vi "mecanum drive.vi"(0 "RobotDriveDevRef":T2={"DevStatus"={"status"=FALSE, "code"=0, "source"=""}, "Motors[]"=[], "Square Inputs"=FALSE, "Max Output"=1.0}, 1 "X Axis":dbl, 2 "Y Axis":dbl, 3 "Z Axis":dbl, 4 "Drive Mode":T1) -> ()   [LabVIEW 2014]
uses:
  <vilib>/Rock Robotics/WPI/RobotDrive/WPI_RobotDriveDevRef.ctl
  <vilib>/Rock Robotics/WPI/MotorControl/WPI_MotorControlDeviceRef.ctl
  <vilib>/Rock Robotics/WPI/MotorControl/WPI_MotorControlType.ctl
  <vilib>/Rock Robotics/SystemInterfaces/Typedef/FPGA_TypedefDigitalModule.ctl
  <vilib>/Rock Robotics/SystemInterfaces/DIO/FPGA_DIOPWMChannel.ctl
  <vilib>/Rock Robotics/WPI/PWM/WPI_PWMDeadband.ctl
  <vilib>/Rock Robotics/WPI/CAN/Jaguar/SubVIs/WPI_CANJaguar_ControlMode.ctl
  <vilib>/Rock Robotics/WPI/CAN/TalonSRX/WPI_CANTalonSRX_APIControlMode.ctl
  <vilib>/Rock Robotics/WPI/PWM/WPI_PWMTransform_ConPane.ctl
  typedefs/mecanum drive mode.ctl
  <vilib>/Rock Robotics/WPI/RobotDrive/WPI_RobotDriveArcadeDrive_Standard(NoSaturation).vi
  <vilib>/Rock Robotics/WPI/RobotDrive/WPI_RobotDriveMecanumDrive_Cartesian.vi
  <vilib>/Rock Robotics/WPI/RobotDrive/WPI_RobotDriveMecanumDrive_Polar.vi
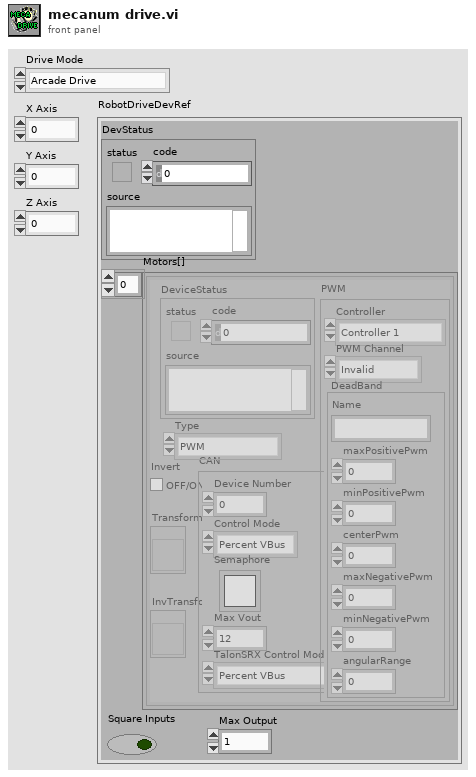
[diagram p1: front panel]
types:
  T1 = typedef "mecanum drive mode.ctl" = enum16{"Arcade Drive", "Left/Right X/Y Control", "Mecanum Cartesian", "Mecanum Cartesian Spin", "Mecanum Polar", "Mecanum Polar Spin"}
  T2 = typedef "WPI_RobotDriveDevRef.ctl" = cluster{"DevStatus":errorcluster, "Motors[]":T3[], "Square Inputs":bool, "Max Output":dbl}
  T3 = typedef "WPI_MotorControlDeviceRef.ctl" = cluster{"DeviceStatus":errorcluster, "Type":T4, "PWM":cluster{"Controller":T5, "PWM Channel":T6, "DeadBand":T7}, "CAN":cluster{"Device Number":u8, "Control Mode":T8, "Semaphore":T9, "Max Vout":dbl, "TalonSRX Control Mode":T10}, "Invert":bool, "TransformRef":T11, "InvTransformRef":T11}
  T4 = typedef "WPI_MotorControlType.ctl" = enum16{"PWM", "CAN", "CANTalonSRX"}
  T5 = typedef "FPGA_TypedefDigitalModule.ctl" = enum16{"Controller 1"}
  T6 = typedef "FPGA_DIOPWMChannel.ctl" = enum8{"PWM 0", "PWM 1", "PWM 2", "PWM 3", "PWM 4", "PWM 5", "PWM 6", "PWM 7", "PWM 8", "PWM 9", "PWM MXP 0", "PWM MXP 1", "PWM MXP 2", "PWM MXP 3", "PWM MXP 4", "PWM MXP 5", "PWM MXP 6", "PWM MXP 7", "PWM MXP 8", "PWM MXP 9", "Invalid"}
  T7 = typedef "WPI_PWMDeadband.ctl" = cluster{"Name":string, "maxPositivePwm":i32, "minPositivePwm":i32, "centerPwm":i32, "maxNegativePwm":i32, "minNegativePwm":i32, "angularRange":u16}
  T8 = typedef "WPI_CANJaguar_ControlMode.ctl" = enum8{"Percent VBus", "Current", "Speed", "Position", "Voltage"}
  T9 = typedef "Semaphore RefNum" = refnum<k1>
  T10 = typedef "WPI_CANTalonSRX_APIControlMode.ctl" = enum8{"Percent VBus", "Speed", "Position", "Slave", "Unchanged / Invalid"}
  T11 = typedef "WPI_PWMTransform_ConPane.ctl" = refnum<vi>
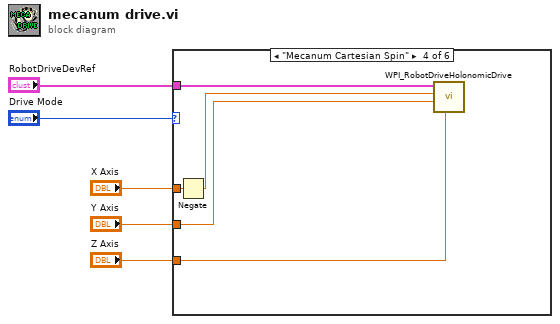
[diagram p0: block diagram]
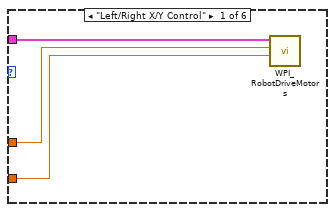
[diagram p2: hidden frame]
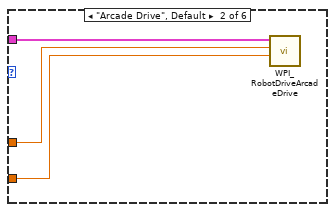
[diagram p3: hidden frame]
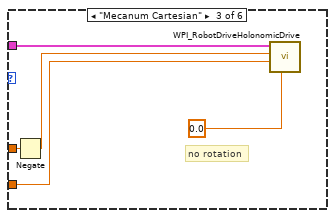
[diagram p4: hidden frame]
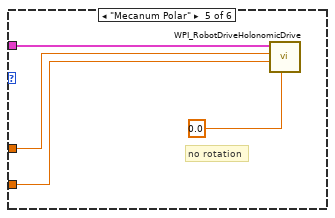
[diagram p5: hidden frame]
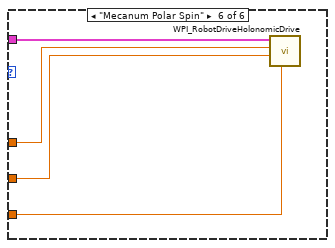
[diagram p6: hidden frame]
diagram:
  n1 = case shown="\"Mecanum Cartesian Spin\"" "Drive Mode" {
    tunnel: "RobotDriveDevRef" -> [w8 w11 w16 w21 w25 w29]
    tunnel: "X Axis" -> [w7 w10 w15 w20 w24 w28]
    tunnel: "Y Axis" -> [w6 w9 w14 w19 w23 w27]
    tunnel: "Z Axis" -> [_ _ _ w18 _ w26]
    frame "Left/Right X/Y Control" {
      n2 = call <vilib>:"WPI_RobotDriveMotors.vi"("RightSpeed"=w6, "LeftSpeed"=w7, "RobotDriveDevRef"=w8) -> ()  [unwired: 6 in, 3 out]
    }
    frame "Arcade Drive", Default {
      n3 = call-poly <vilib>:"WPI_RobotDriveArcadeDrive.vi"("Y axis value"=w9, "X axis value"=w10, "RobotDriveDevRef"=w11) -> ()  [unwired: 6 in, 3 out]
    }
    frame "Mecanum Cartesian" {
      # "no rotation"
      n4 = Negate(x=w15) -> (-x=w12:dbl)
      n5 = call-poly <vilib>:"WPI_RobotDriveHolonomicDrive.vi"("Rotation"=0.0, "Y"=w14, "X"=w12, "RobotDriveDevRef"=w16) -> ()  [unwired: 5 in, 3 out]
    }
    frame "Mecanum Cartesian Spin" {
      n6 = Negate(x=w20) -> (-x=w17:dbl)
      n7 = call-poly <vilib>:"WPI_RobotDriveHolonomicDrive.vi"("Rotation"=w18, "Y"=w19, "X"=w17, "RobotDriveDevRef"=w21) -> ()  [unwired: 5 in, 3 out]
    }
    frame "Mecanum Polar" {
      # "no rotation"
      n8 = call-poly <vilib>:"WPI_RobotDriveHolonomicDrive.vi"("Rotation"=0.0, "Direction"=w23, "Magnitude"=w24, "RobotDriveDevRef"=w25) -> ()  [unwired: 5 in, 3 out]
    }
    frame "Mecanum Polar Spin" {
      n9 = call-poly <vilib>:"WPI_RobotDriveHolonomicDrive.vi"("Rotation"=w26, "Direction"=w27, "Magnitude"=w28, "RobotDriveDevRef"=w29) -> ()  [unwired: 5 in, 3 out]
    }
  }
